vi "GetDistanceFromAngles.vi"(10 "Next Point":dbl, 11 "Current Point":dbl) -> (2 "Distance To Go":dbl, 3 "New Point":dbl)   [LabVIEW 2015]
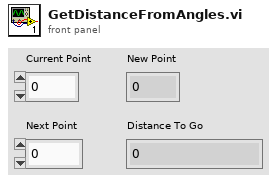
[diagram p1: front panel]
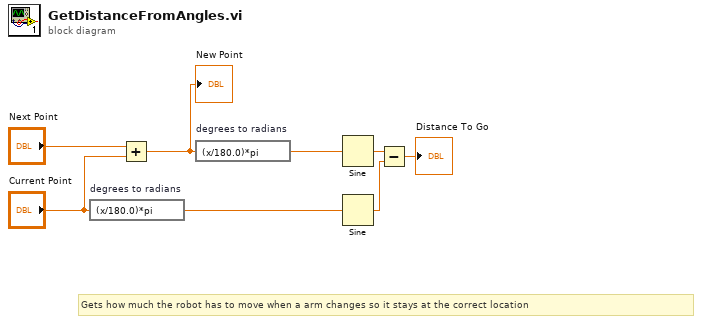
[diagram p0: block diagram]
diagram:
  # "Gets how much the robot has to move when a arm changes so it stays at the correct location"
  n1 = expression code="(x/180.0)*pi" "degrees to radians"("Current Point") -> (w5:dbl)
  n2 = Add(x="Next Point", y="Current Point") -> (x+y=w3:dbl)
  "New Point" <- w3
  n3 = expression code="(x/180.0)*pi" "degrees to radians"(w3) -> (w4:dbl)
  n4 = Sine(x=w4) -> (sin(x)=w6:dbl)
  n5 = Sine(x=w5) -> (sin(x)=w7:dbl)
  n6 = Subtract(x=w6, y=w7) -> (x-y=→"Distance To Go":dbl)
